vi "test_Basic Deployment.vi"(8 "error in (no error)":errorcluster, 11 "TestCase in":refnum<class "Telemetry System Tests.lvclass">=refnum) -> (0 "error out":errorcluster, 3 "TestCase out":refnum<class "Telemetry System Tests.lvclass">)   [LabVIEW 2026, in "Telemetry System Tests.lvclass"]
uses:
  Telemetry System Tests.lvclass
  Telemetry System Tests.lvclass/Telemetry System Tests.ctl
  16843a54-b407-40ab-9d94-4c25adff9086.vi
  <vilib>/NI/VeriStand Custom Device Testing Tools/VeriStandTestUtilities/TargetPlatform.ctl
  <vilib>/NI/VeriStand Custom Device Testing Tools/VeriStandTestUtilities/VeriStandTestUtilities.lvlib
  <vilib>/NI/VeriStand Custom Device Testing Tools/VeriStandTestUtilities/ChassisInformation.ctl
  <vilib>/NI/VeriStand Custom Device Testing Tools/VeriStandTestUtilities/TargetInformation.ctl
  <vilib>/NI/VeriStand Custom Device Testing Tools/VeriStandTestUtilities/SystemDefinitionInformation.ctl
panel:
  out "System Definition Information":T1
  out "Active Configuration":T4
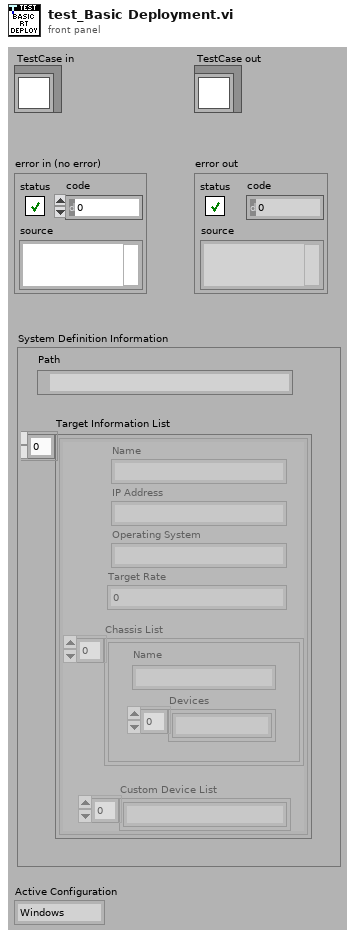
[diagram p1: front panel]
types:
  T1 = typedef "VeriStandTestUtilities.lvlib/SystemDefinitionInformation.ctl" = cluster{"Path":path, "Target Information List":T2[]}
  T2 = typedef "VeriStandTestUtilities.lvlib/TargetInformation.ctl" = cluster{"Name":string, "IP Address":string, "Operating System":string, "Target Rate":dbl, "Chassis List":T3[], "Custom Device List":string[]}
  T3 = typedef "VeriStandTestUtilities.lvlib/ChassisInformation.ctl" = cluster{"Name":string, "Devices":string[]}
  T4 = typedef "VeriStandTestUtilities.lvlib/TargetPlatform.ctl" = enum16{"Windows", "Linux64CRIO", "Linux64PXI", "LinuxARM", "PharLap"}
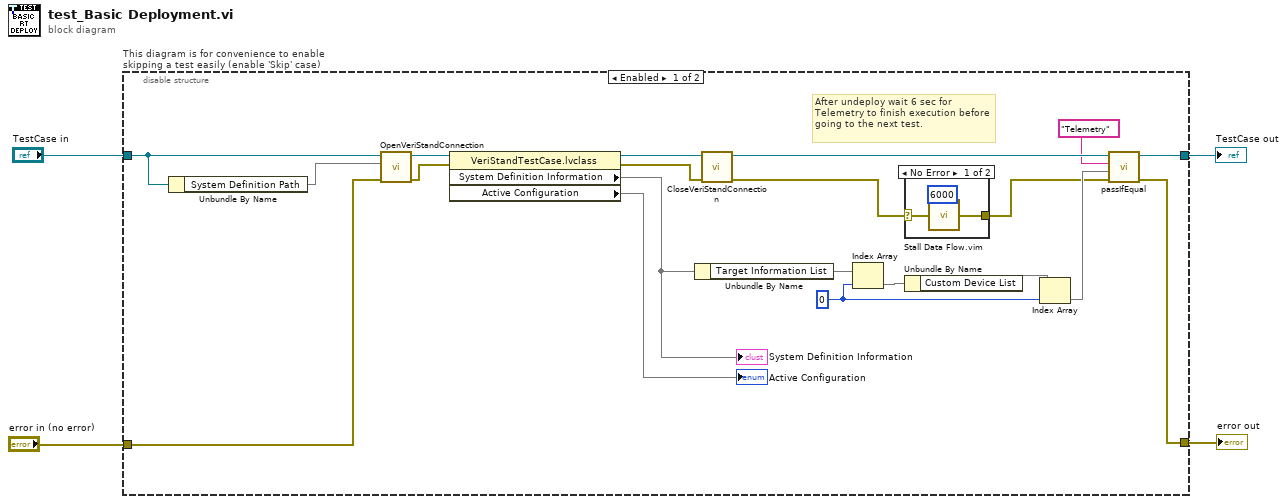
[diagram p0: block diagram]
diagram:
  n1 = disable-structure "This diagram is for convenience to enable skipping a test easily (enable 'Skip' case)" shown="Enabled" {
    disable-tunnel: "TestCase in" -> [w9 w32]
    disable-tunnel: [w10 w30] -> w1
    disable-tunnel: [w5 w31] -> w3
    disable-tunnel: "error in (no error)" -> [w24 w29]
    frame Enabled {
      w14 = 0 ("index")
      # "After undeploy wait 6 sec for Telemetry to finish execution before going to the next test."
      n2 = Unbundle By Name(w9) -> ("System Definition Path"=w8)
      n3 = call-dynamic "OpenVeriStandConnection.vi"("error in (no error)"=w24, "System Definition File"=w8, "VeriStand Test Case in"=w9) -> ("error out"=w20:errorcluster, "VeriStand Test Case out"=w23:refnum<class "VeriStandTestCase.lvclass">)  [unwired: 6 in, 1 out]
      n4 = property class="VeriStandTestCase.lvclass"(reference=w23, error in=w20) -> (reference out=w22:refnum<class "VeriStandTestCase.lvclass">, error out=w18:errorcluster, "System Definition Information"=w19, "Active Configuration"=→"Active Configuration")
      "System Definition Information" <- w19
      n5 = Unbundle By Name(w19) -> ("Target Information List"=w17)
      n6 = call-dynamic "CloseVeriStandConnection.vi"("error in (no error)"=w18, "VeriStand Test Case in"=w22) -> ("error out"=w7:errorcluster, "VeriStand Test Case out"=w13:refnum<class "VeriStandTestCase.lvclass">)  [unwired: 8 in]
      n7 = Index Array(array=w17, index=w14) -> (element=w16)
      n8 = case shown="No Error" w7 {
        selector: w7 -> [w27 w28]
        tunnel: [w25 w28] -> w6
        frame No Error {
          n9 = call "Stall Data Flow.vim"("value in"=w27, "milliseconds to wait"=u32 6000) -> ("value out"=w25:errorcluster)  [unwired: 1 out]
        }
        frame Error {
        }
      }
      n10 = Unbundle By Name(w16) -> ("Custom Device List"=w15)
      n11 = Index Array(array=w15, index=w14) -> (element=w12)
      n12 = call-dynamic "passIfEqual.vi"("error in (no error)"=w6, "y"=w12, "x"="Telemetry" ("element"), "TestCase in"=w13) -> ("error out"=w5:errorcluster, "TestCase out"=w10:refnum<class "Telemetry System Tests.lvclass">)  [unwired: 6 in]
    }
    frame Disabled {
      # "skip test result while test is under development"
      n13 = call <vilib>:"skip.vi"("error in (no error)"=w29, "TestCase in"=w32) -> ("error out"=w31:errorcluster, "TestCase out"=w30:refnum<class "Telemetry System Tests.lvclass">)  [unwired: 8 in]
    }
  }
  "error out" <- w3
  "TestCase out" <- w1
